vi "FPGA Main R2 AB JC KV.vi"() -> ()   [LabVIEW 2018]
uses:
  <vilib>/rvi/Emulation/niFpgaGetClockAttributes.vi
  <vilib>/rvi/Emulation/niFpgaSctlEmulationGetInTimedLoop.vi
  <vilib>/rvi/Emulation/niFpgaEmulationReportErrorSimple.vi
  <vilib>/rvi/eio/common/nirviEmuTemplateMethod_errors.vi
  <vilib>/rvi/Emulation/niFpgaProcessEmulError.vi
  <vilib>/rvi/interface/RandomDataEmulation/niFpgaRandomDataHandleErrors.vi
  <vilib>/rvi/Emulation/niFpgaCriticalErrorInLSC.vi
  <vilib>/rvi/Analysis/control/PID/SubVIs/niFpgaPID_PIWrapper.vi
  <vilib>/eio/EIONode/EIONode.xnode
  <vilib>/rvi/DataTransferAndStorage/Container/XNode/niFpgaContainer.xnode
  <vilib>/rvi/interface/RandomDataEmulation/nirviRandomDataFpgaReadWriteTemplate.vi
panel:
  in  "Manual/PID":bool
  out "PID Error (V)":sgl
  out "PID Output (V)":u16
  in  "Output Limits":cluster{"Vmax":sgl, "Vmin":sgl}
  in  "PID Gains":cluster{"Kp":sgl, "Ki":sgl}
  out "Capacitance\nProbe (V)":u16
  out "Coil Back \nEMF (V)":u16
  in  "Control Loop \nRate (uSec)":u32
  in  "Sensor Loop \nRate (uSec)":u32
  in  "VC Command (V)":u16
  in  "Amplifier On/Off":bool
  # "Controls"
  # "PID Settings"
  # "Sensors"
  # "Loop Rates"
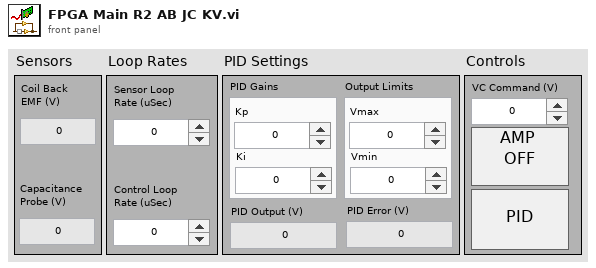
[diagram p1: front panel]
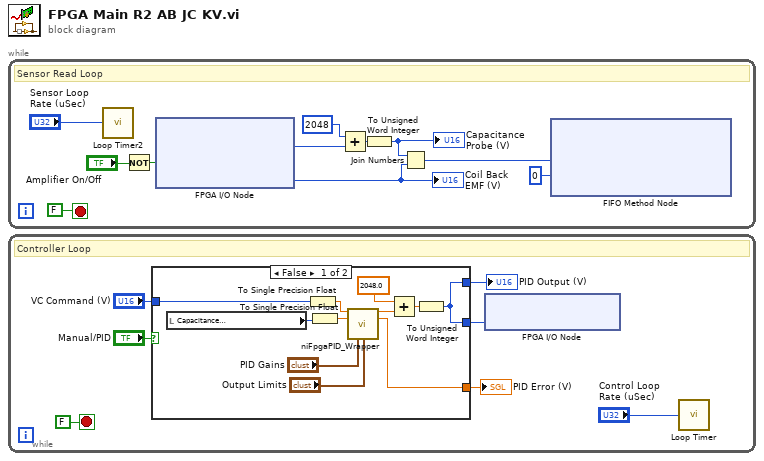
[diagram p0: block diagram]
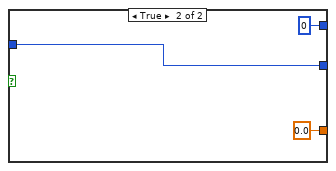
[diagram p2: hidden frame]
diagram:
  n1 = while {
    stop <- FALSE stop-if-true
    # "Sensor Read Loop"
    n2 = call "Loop Timer2"("Count(uSec)"="Sensor Loop \nRate (uSec)") -> ()  [unwired: 1 out]
    n3 = Not(x="Amplifier On/Off") -> (.not. x?=w1:bool)
    n4 = xnode "FPGA I/O Node"("ConnectorA/DIO9"=w1) -> ("ConnectorC/AI0"=w10:i16, "ConnectorA/AI1"=w6:u16)  [unwired: 3 in, 3 out]
    "Coil Back \nEMF (V)" <- w6
    n5 = Add(x=i16 2048, y=w10) -> (x+y=w11:i16)
    n6 = To Unsigned Word Integer(number=w11) -> (unsigned 16bit integer=w5:u16)
    "Capacitance\nProbe (V)" <- w5
    n7 = Join Numbers(hi=w5, lo=w6) -> ((hi.lo)=w7:u32)
    n8 = xnode ("FIFO Method Node")("Element"=w7, "Timeout"=0) -> ()  [unwired: 1 in, 2 out]
  }
  n9 = while {
    stop <- FALSE stop-if-true
    # "Controller Loop"
    n10 = case shown="False" "Manual/PID" {
      tunnel: "VC Command (V)" -> [w28 w30]
      tunnel: [w19 u16 0] -> w16
      tunnel: [w22 sgl 0.0 ("error")] -> w15
      tunnel: [w19 w30] -> w13
      frame False {
        n11 = local read "Capacitance\nProbe (V)"() -> (w26:u16)
        n12 = To Single Precision Float(number=w28) -> (single precision float=w27:sgl)
        n13 = To Single Precision Float(number=w26) -> (single precision float=w29:sgl)
        n14 = call-poly <vilib>:"niFpgaPID_Wrapper.vi"("setpoint"=w27, "process variable"=w29, "gains"="PID Gains", "output range"="Output Limits") -> ("output"=w21:sgl, "error"=w22:sgl)  [unwired: 9 in, 1 out]
        n15 = Add(x=sgl 2048.0, y=w21) -> (x+y=w23:sgl)
        n16 = To Unsigned Word Integer(number=w23) -> (unsigned 16bit integer=w19:u16)
      }
      frame True {
      }
    }
    "PID Output (V)" <- w16
    "PID Error (V)" <- w15
    n17 = xnode "FPGA I/O Node"("ConnectorA/AO1"=w13) -> ()  [unwired: 1 in, 1 out]
    n18 = call "Loop Timer"("Count(uSec)"="Control Loop \nRate (uSec)") -> ()  [unwired: 1 out]
  }
